vi "Get Inline Transmit Transfer Groups.vi"(11 "Plugin in":refnum<class "Plugin.lvclass">) -> (2 "Inline Tx Transfer Groups":refnum<class "Transfer Group.lvclass">[](array[class]), 3 "Plugin out":refnum<class "Plugin.lvclass">)   [LabVIEW 2017, in "Data Sharing Framework Core.lvlib" / "Data Sharing Framework Engine.lvlib" / "Plugin.lvclass"]
uses:
  Plugin.lvclass
  Transfer Group/Transfer Group.lvclass
  Plugin.lvclass/Plugin.ctl
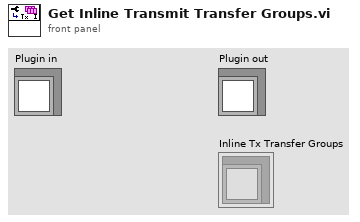
[diagram p1: front panel]
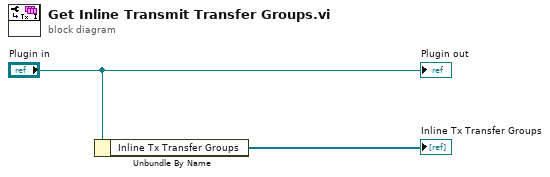
[diagram p0: block diagram]
diagram:
  n1 = Unbundle By Name("Plugin in") -> ("Inline Tx Transfer Groups"=→"Inline Tx Transfer Groups":refnum<class "Transfer Group.lvclass">[])
  "Plugin out" <- "Plugin in"
